vi "Write Config Settings.vi"(8 "error in (no error)":errorcluster, 9 "Config Settings":T1={"Application Settings"={"Simulation"=FALSE}, "Main Settings"={"Simulation"=FALSE, "Signal scaling"=[], "ESR scaling"=[], "num readings to average"=[], "ESR alarm threshhold (%)"=[], "UseDummyVrms"=FALSE, "Dummy Vrms"=0.0, "Inverter Database File"=path "", "default Inverter (name)"=[]}, "DAQ Settings"={"Simulation"=FALSE, "Initial ErrReporting setting"=0, "Initial Measurement settings"={"Data Rate 9775"=3.0, "Data Rate 9215"=1200000.0, "Samples RMS 9215"=480000, "Samples RMS 9775"=3}, "Acquisition mode"=enum."3phase", "DemoMode"=FALSE, "RIO Device"=""}, "LogEngine Settings"={"Simulation"=FALSE, "TDMS_FolderPath"="", "CSV_FolderPath"="", "TDMS_FileName_Prefix"="", "CSV_FileName_Prefix"="", "TDMS_LogDuration(s)"=0.0, "CSV_LogDuration(s)"=0.0}} {"Main Settings"."Dummy Vrms" format="%.2g"; "DAQ Settings"."Initial ErrReporting setting" items=["DONTPRINT", "PRINTWARNINGS", "PRINTFATAL", "PRINTALL"]}, 10 "ConfigFile":path, 11 "Config in":refnum<class "Config.lvclass">) -> (0 "error out":errorcluster, 2 "ConfigFile out":path, 3 "Config out":refnum<class "Config.lvclass">)   [LabVIEW 2019, in "Config.lvclass"]
doc: "Developed by Kevin Thompson\nkevin@thompsonengineering.net\n\nCopyright 2018-2020\nThompson Engineering, LLC"
uses:
  Config.lvclass
  DataTypes/Config Settings.ctl
  Application/DataTypes/Settings--cluster.ctl
  Main/DataTypes/Settings--cluster.ctl
  Main/support/Data Algorithms/subvis/DataTypes/Gain control.ctl
  Main/support/Data Algorithms/subvis/DataTypes/ESR scaling--cluster.ctl
  DAQ_Engine/DataTypes/Settings--cluster.ctl
  Common/DataTypes/Measurement Config--cluster.ctl
  Common/DataTypes/Acquisition Mode--cluster.ctl
  Log_Engine/DataTypes/Settings--cluster.ctl
  Config.lvclass/Config.ctl
  Accessors/Set Application Settings.vi
  Accessors/Set Main Settings.vi
  Accessors/Set LogEngine Settings.vi
  Accessors/Set DAQ Settings.vi
  Application/Application.lvclass
  DAQ_Engine/DAQ_Engine.lvclass
  Log_Engine/Log_Engine.lvclass
  Main/Main.lvclass
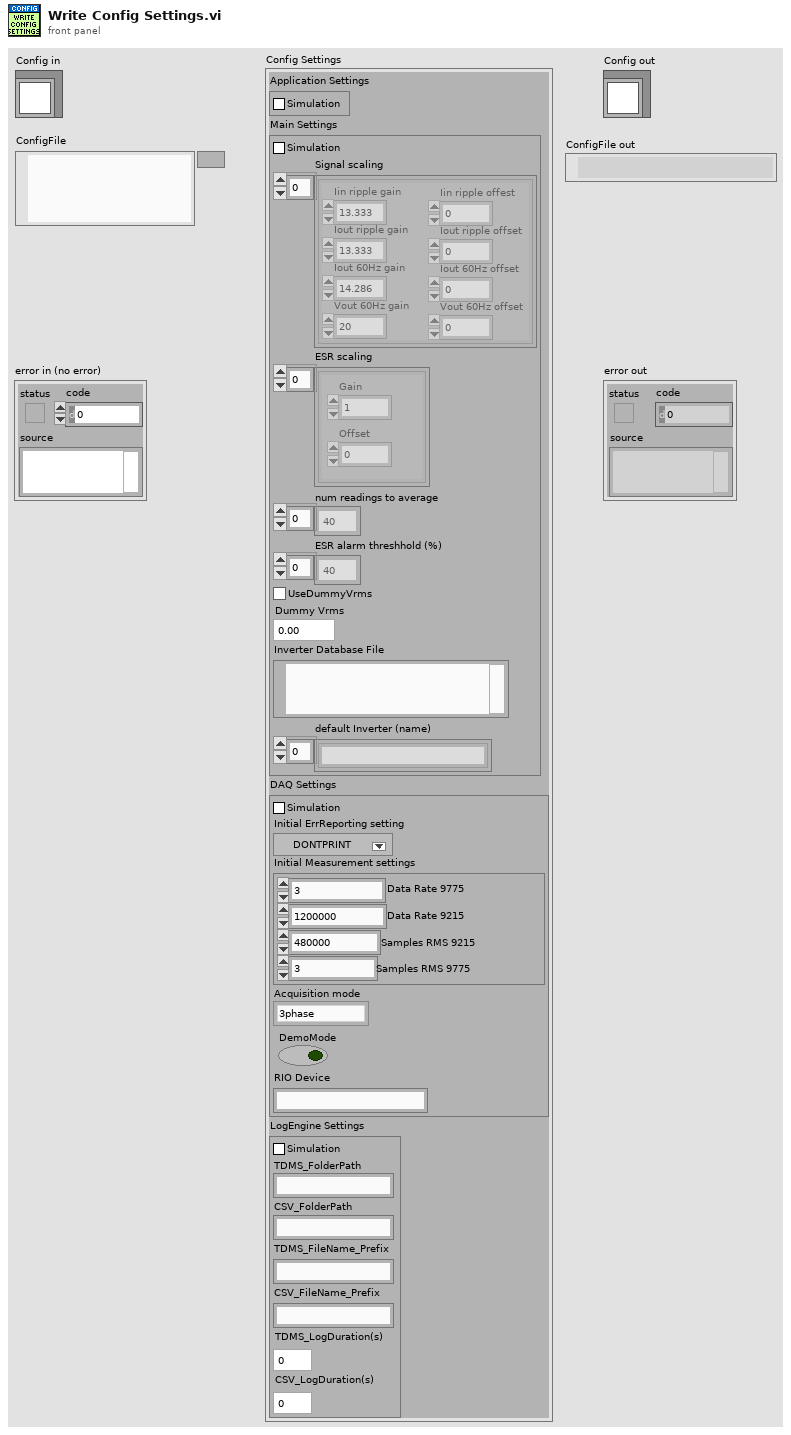
[diagram p1: front panel]
types:
  T1 = typedef "Config.lvclass/Config Settings.ctl" = cluster{"Application Settings":T2, "Main Settings":T3, "DAQ Settings":T6, "LogEngine Settings":T9}
  T2 = typedef "Application.lvclass/Settings--cluster.ctl" = cluster{"Simulation":bool}
  T3 = typedef "Main.lvclass/Settings--cluster.ctl" = cluster{"Simulation":bool, "Signal scaling":T4[], "ESR scaling":T5[], "num readings to average":i32[], "ESR alarm threshhold (%)":i32[], "UseDummyVrms":bool, "Dummy Vrms":dbl, "Inverter Database File":path, "default Inverter (name)":string[]}
  T4 = typedef "Main.lvclass/Gain control.ctl" = cluster{"Iin ripple gain":dbl, "Iout ripple gain":dbl, "Iout 60Hz gain ":dbl, "Vout 60Hz gain ":dbl, "Iin ripple offest":dbl, "Iout ripple offset":dbl, "Iout 60Hz offset":dbl, "Vout 60Hz offset":dbl}
  T5 = typedef "Main.lvclass/ESR scaling--cluster.ctl" = cluster{"Gain":dbl, "Offset":dbl}
  T6 = typedef "DAQ_Engine.lvclass/Settings--cluster.ctl" = cluster{"Simulation":bool, "Initial ErrReporting setting":i32, "Initial Measurement settings":T7, "Acquisition mode":T8, "DemoMode":bool, "RIO Device":string}
  T7 = typedef "Measurement Config--cluster.ctl" = cluster{"Data Rate 9775":dbl, "Data Rate 9215":dbl, "Samples RMS 9215":u32, "Samples RMS 9775":u32}
  T8 = typedef "Acquisition Mode--cluster.ctl" = enum16{"3phase", "Single"}
  T9 = typedef "Log_Engine.lvclass/Settings--cluster.ctl" = cluster{"Simulation":bool, "TDMS_FolderPath":string, "CSV_FolderPath":string, "TDMS_FileName_Prefix":string, "CSV_FileName_Prefix":string, "TDMS_LogDuration(s)":dbl, "CSV_LogDuration(s)":dbl}
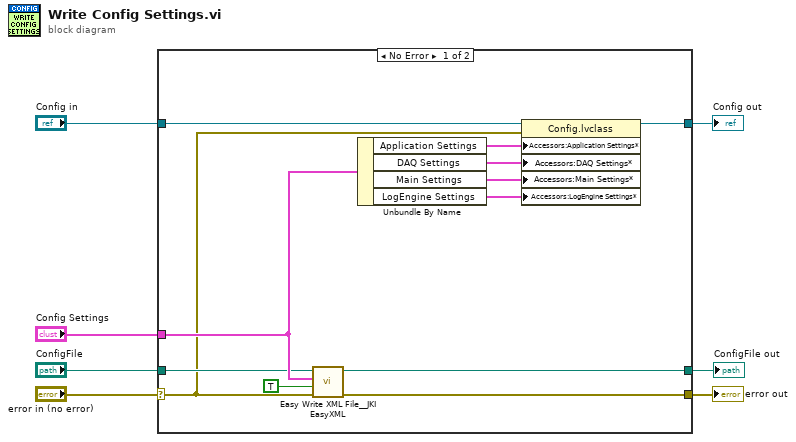
[diagram p0: block diagram]
diagram:
  n1 = case shown="No Error" "error in (no error)" {
    selector: "error in (no error)" -> [w10 w22]
    tunnel: [w9 w22] -> w6
    tunnel: [w18 w21] -> w4
    tunnel: "Config in" -> [w19 w21]
    tunnel: "Config Settings" -> [w13 _]
    tunnel: "ConfigFile" -> [w12 w20]
    tunnel: [w8 w20] -> w1
    frame No Error {
      n2 = call <vilib>:"Easy Write XML File__JKI EasyXML.vi"("error in (no error)"=w10, "Overwrite File? (false)"=TRUE, "LabVIEW Data"=w13, "XML File Path"=w12) -> ("error out"=w9:errorcluster, "XML File Path (duplicate)"=w8:path)  [unwired: 6 in]
      n3 = Unbundle By Name(w13) -> ("Application Settings"=w14:T2, "DAQ Settings"=w17:T6, "Main Settings"=w16:T3, "LogEngine Settings"=w15:T9)
      n4 = property class="Config.lvclass"(reference=w19, error in=w10, "Accessors:Application Settings*"=w14, "Accessors:DAQ Settings*"=w17, "Accessors:Main Settings*"=w16, "Accessors:LogEngine Settings*"=w15) -> (reference out=w18:refnum<class "Config.lvclass">)  [unwired: 1 out]
    }
    frame Error {
    }
  }
  "error out" <- w6
  "Config out" <- w4
  "ConfigFile out" <- w1
